vi "Read_DI_DO_Together.vi"(8 "error in (no error)":errorcluster, 9 "quantity":u16, 10 "starting address":u16, 11 "MB session in":refnum<class "MB_Master.lvclass">) -> (0 "error out":errorcluster, 1 "Coils 2":bool[](array[boolean]), 2 "Coils":bool[](array[boolean]), 3 "MB session out":refnum<class "MB_Master.lvclass">, 5 "Registers":u16[](array[numeric]))   [LabVIEW 2016, in "MB Master.lvlib"]
uses:
  MB Master.lvlib
  MB_Master.lvclass
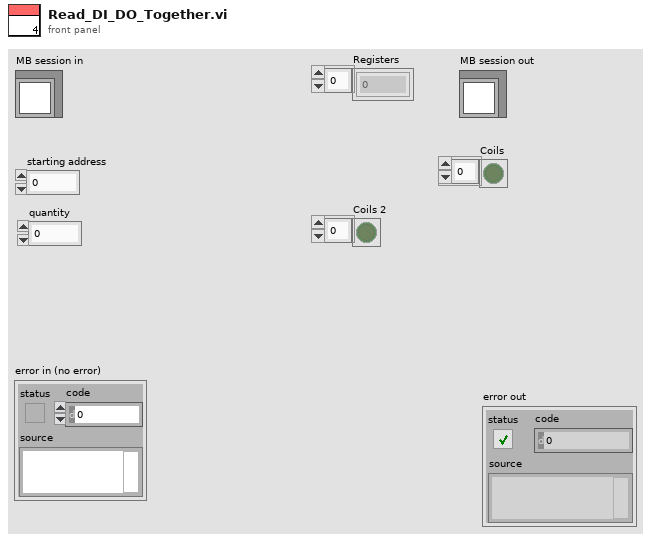
[diagram p1: front panel]
types:
  T1 = typedef "MB Master.lvlib/MB_PDU_Cluster.ctl" = cluster{"Function Code":u8, "Data":u8[], "RTU_DataBytes":i32}
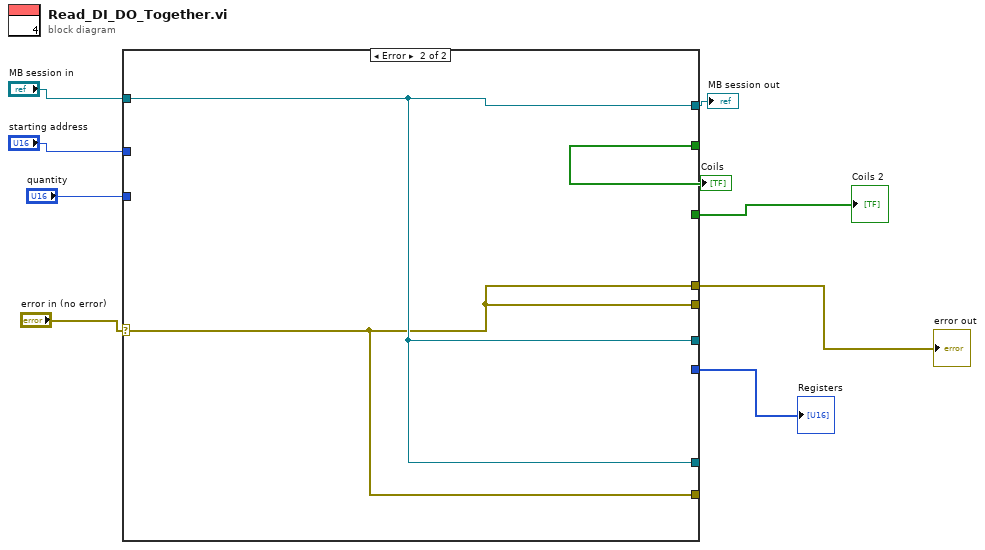
[diagram p0: block diagram]
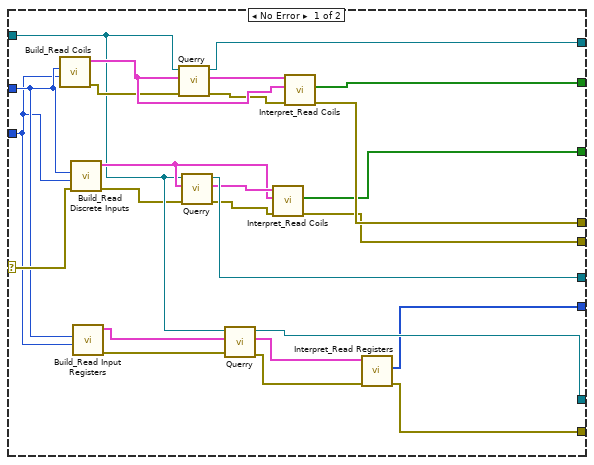
[diagram p2: hidden frame]
diagram:
  n1 = case shown="Error" "error in (no error)" {
    selector: "error in (no error)" -> [w23 w35]
    tunnel: "quantity" -> [w20 _]
    tunnel: "starting address" -> [w21 _]
    tunnel: "MB session in" -> [w19 w36]
    tunnel: [w30 w36] -> w5
    tunnel: [w34 w35] -> w4
    tunnel: [w33 _] -> w3
    tunnel: [w32 w35] -> _
    tunnel: [w31 _] -> w2
    tunnel: [w29 w36] -> _
    tunnel: [w18 w36] -> _
    tunnel: [w11 w35] -> _
    tunnel: [w10 _] -> w1
    frame No Error {
      n2 = call "Build_Read Coils.vi"("quantity"=w20, "starting address"=w21) -> ("error out"=w24:errorcluster, "MB_PDU"=w26:T1)  [unwired: 8 in]
      n3 = call "Build_Read Discrete Inputs.vi"("error in (no error)"=w23, "quantity"=w20, "starting address"=w21) -> ("error out"=w16:errorcluster, "MB_PDU"=w22:T1)  [unwired: 7 in]
      n4 = call "Build_Read Input Registers.vi"("quantity"=w20, "starting address"=w21) -> ("error out"=w15:errorcluster, "MB_PDU"=w14:T1)  [unwired: 8 in]
      n5 = call-dynamic "Querry.vi"("error in (no error)"=w24, "PDU_req"=w26, "MB_Master in"=w19) -> ("error out"=w25:errorcluster, "PDU_resp"=w27:T1, "MB_Master out"=w30:refnum<class "MB_Master.lvclass">)  [unwired: 6 in]
      n6 = call-dynamic "Querry.vi"("error in (no error)"=w16, "PDU_req"=w22, "MB_Master in"=w19) -> ("error out"=w17:errorcluster, "PDU_resp"=w28:T1, "MB_Master out"=w29:refnum<class "MB_Master.lvclass">)  [unwired: 6 in]
      n7 = call-dynamic "Querry.vi"("error in (no error)"=w15, "PDU_req"=w14, "MB_Master in"=w19) -> ("error out"=w12:errorcluster, "PDU_resp"=w13:T1, "MB_Master out"=w18:refnum<class "MB_Master.lvclass">)  [unwired: 6 in]
      n8 = call "Interpret_Read Coils.vi"("error in (no error)"=w17, "MB_PDU_req in"=w22, "MB_PDU_resp in"=w28) -> ("error out"=w32:errorcluster, "Coils"=w31:bool[])  [unwired: 7 in]
      n9 = call "Interpret_Read Coils.vi"("error in (no error)"=w25, "MB_PDU_req in"=w26, "MB_PDU_resp in"=w27) -> ("error out"=w34:errorcluster, "Coils"=w33:bool[])  [unwired: 7 in]
      n10 = call "Interpret_Read Registers.vi"("error in (no error)"=w12, "MB_PDU_resp in"=w13) -> ("error out"=w11:errorcluster, "Registers"=w10:u16[])  [unwired: 8 in]
    }
    frame Error {
    }
  }
  "MB session out" <- w5
  "Coils" <- w3
  "error out" <- w4
  "Coils 2" <- w2
  "Registers" <- w1
